vi "Read Time Measurement Requested.vi"(8 "error in (no error)":errorcluster, 11 "Measurement in":refnum<class "Measurement.lvclass">) -> (0 "error out":errorcluster, 2 "Time Measurement Requested":timestamp, 3 "Measurement out":refnum<class "Measurement.lvclass">)   [LabVIEW 2016, in "Measurement Actor.lvlib" / "Measurement.lvclass"]
uses:
  Measurement.lvclass
  Measurement.lvclass/Measurement.ctl
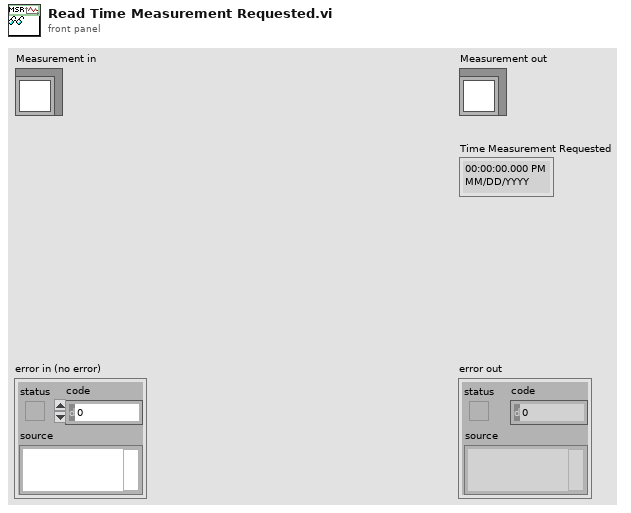
[diagram p1: front panel]
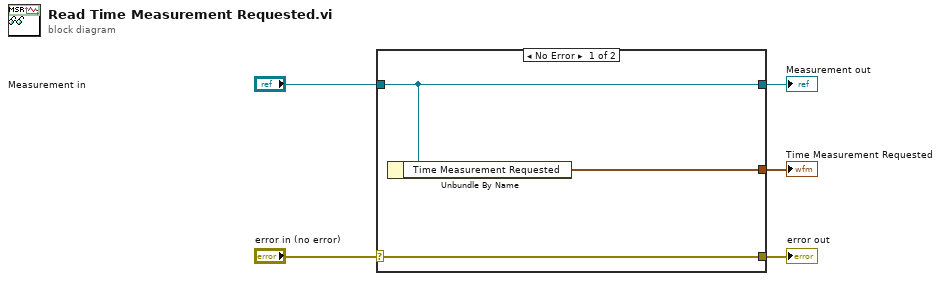
[diagram p0: block diagram]
diagram:
  n1 = case shown="No Error" "error in (no error)" {
    selector: "error in (no error)" -> [w8 w9]
    tunnel: [w8 w9] -> w4
    tunnel: [w7 w10] -> w2
    tunnel: "Measurement in" -> [w7 w10]
    tunnel: [w6 _] -> w1
    frame No Error {
      n2 = Unbundle By Name(w7) -> ("Time Measurement Requested"=w6:timestamp)
    }
    frame Error {
    }
  }
  "error out" <- w4
  "Measurement out" <- w2
  "Time Measurement Requested" <- w1
